vi "Kinect Demo.vi"() -> ()   [LabVIEW 2011]
uses:
  <vilib>/Utility/sysdir.llb/System Directory Type.ctl
  <vilib>/Platform/TimedLoop/XDataNode/XDataNode.xnode
  <vilib>/Platform/TimedLoop/XDataNode/nitl_modes.ctl
  <vilib>/Platform/TimedLoop/XDataNode/XDNodeRunTimeDep.lvlib
  <vilib>/Platform/TimedLoop/XDataNode/wakeup.ctl
  <vilib>/Platform/TimedLoop/XDataNode/timing_clust.ctl
  <vilib>/vision/NI_Vision_Development_Module.lvlib
panel:
  in  "Operation":T1(ring)=enum."Open"
  in  "Display Type":T2(ring)=enum."Baseline"
  in  "Post Extraction Limit":cluster{dbl, dbl}(slide)={0.0, 6291.456} scale=-3000.0..3000.0
  in  "stop 2":bool
  in  "# Frames in Average":i32=100
  in  "Start":bool
  in  "Zero Out Baseline":bool
  in  "Median Filter Size":i32=5 min=0 max=7
  in  "Divisor":sgl=0.5 min=0 max=1 step=0.1
  in  "name or relative path":string="Mouse Test"
  in  "Distance to Camera Visible":cluster{dbl, dbl}(slide)={0.0, 6291.456} scale=-32768.0..32768.0
  in  "Status":string
  out "Frame Display":T3(plugin-control)
  out "Image":T3(plugin-control)
  in  "stop":bool
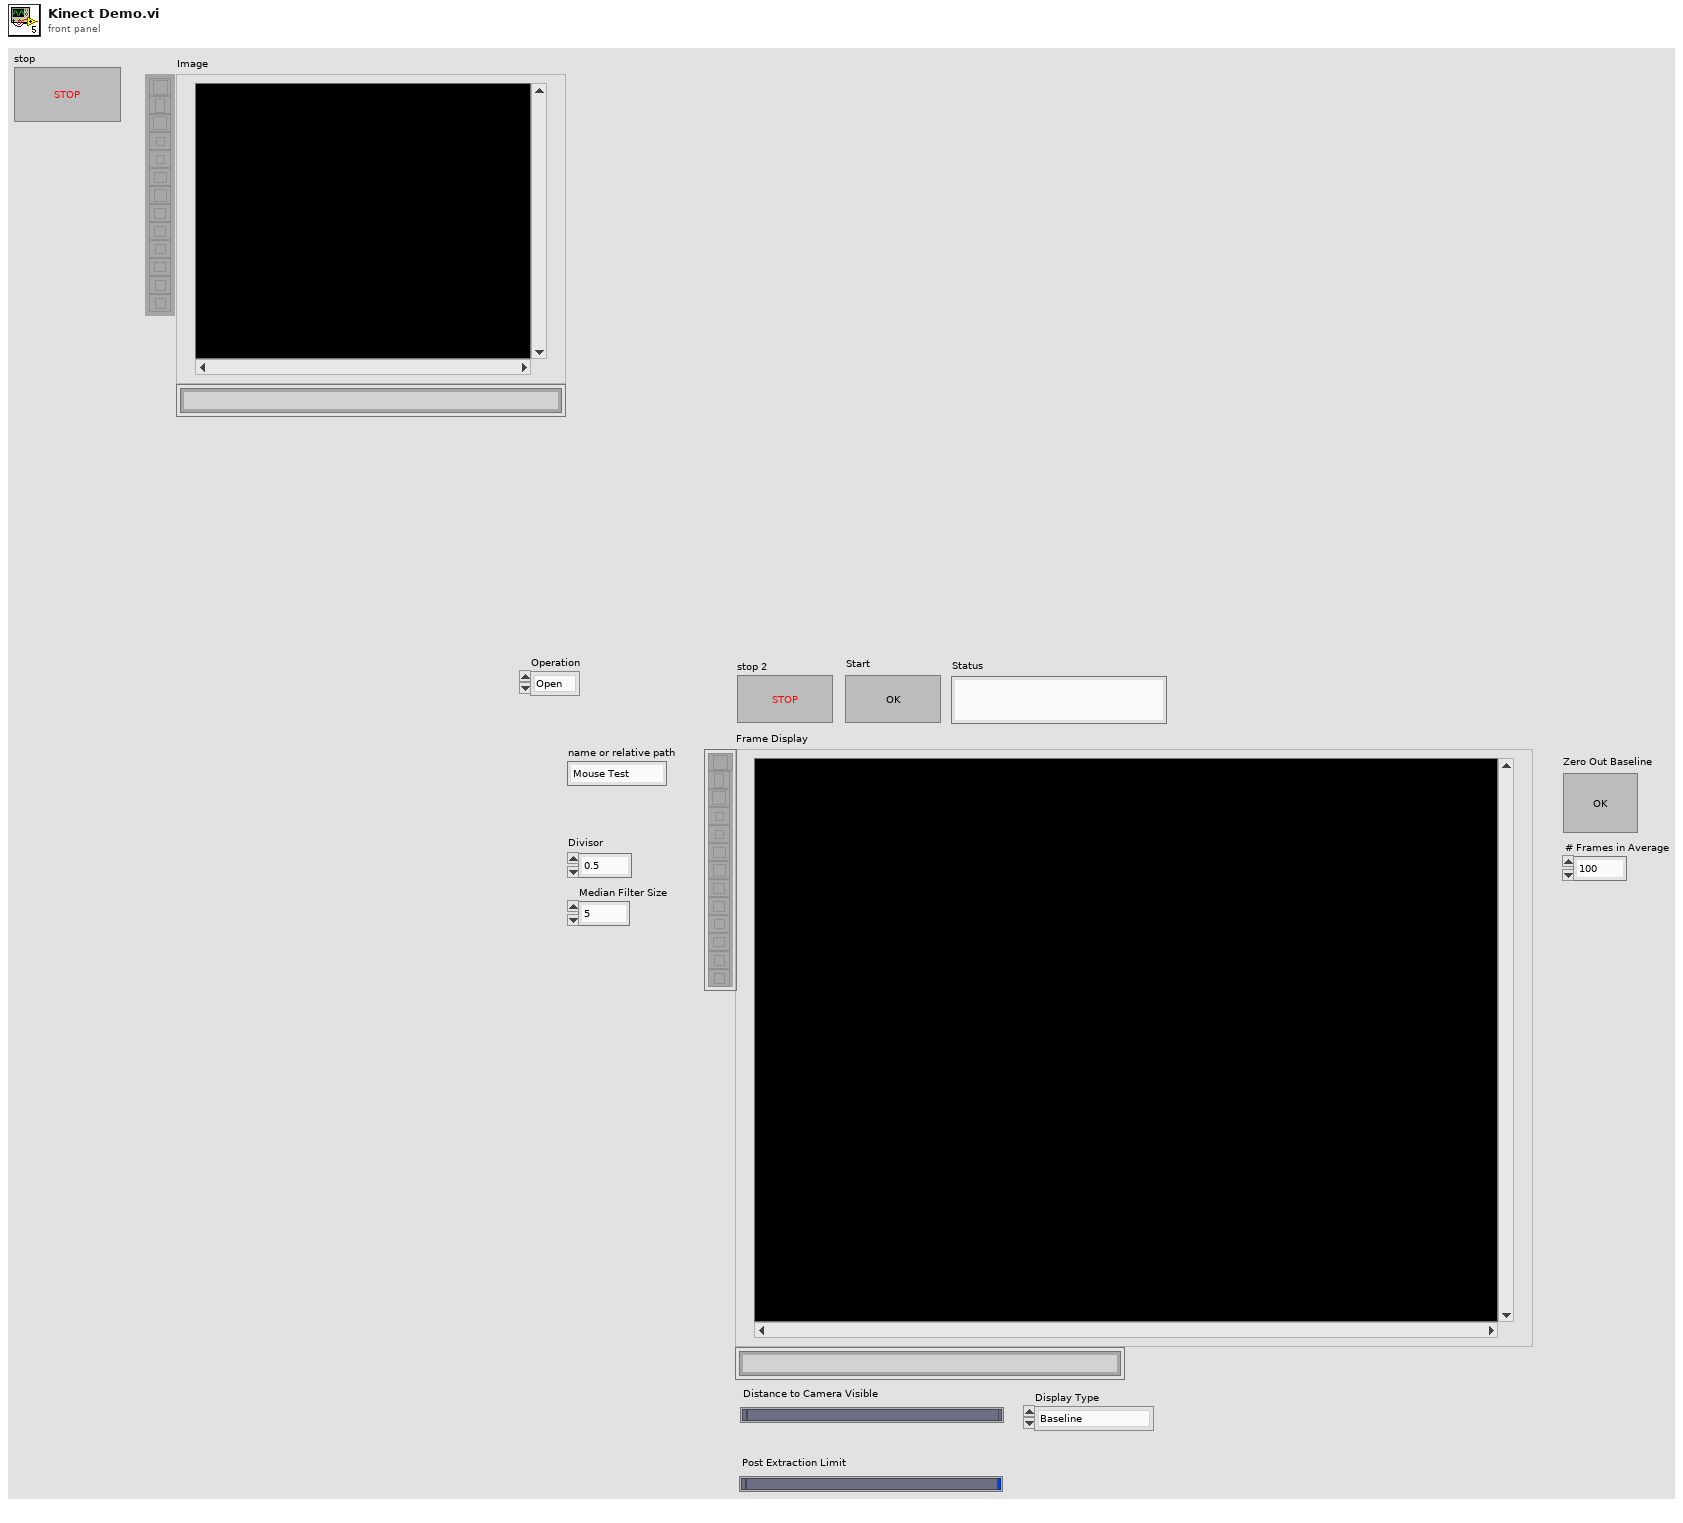
[diagram p1: front panel]
types:
  T1 = enum32{"AutoM", "Close", "Dilate", "Erode", "Gradient", "Gradient in", "Gradient out", "HitMiss", "Open", "PClose", "POpen", "Thick", "Thin"}
  T2 = enum16{"Raw Image", "Baseline", "Baseline Extracted"}
  T3 = typedef "IMAQ Image.ctl" = refnum<image>
  T4 = typedef "System Directory Type.ctl" = i32
  T5 = enum16{"Record", "Idle", "Acquire Background", "Stop"}
  T6 = typedef "XDNodeRunTimeDep.lvlib/timing_clust.ctl" = cluster{"Expected End [f-1]":u64, "Actual End [f-1]":u64, "Finished Late? [f-1]":bool, "Expected End [i-1]":u64, "Actual End [i-1]":u64, "Finished Late? [i-1]":bool, "Expected Start [i]":u64, "Actual Start [i]":u64, "Expected Start [f]":u64, "Actual Start [f]":u64, "Source Name":string, "Structure Name":string, "Period":i64, "Deadline":i64, "Offset":i64, "Start":i64, "Priority":i32, "Timeout":i32, "Mode":T7, "Wakeup Reason":T8, "Error":errorcluster, "Source Type":string, "Secondary Source Type":string, "Global End Time":u64, "Global Start Time":u64, "Frame Duration":u64, "Iteration Duration":u64, "Assigned CPU":i32, "I/O Scan Engine Mode":u32}
  T7 = typedef "XDNodeRunTimeDep.lvlib/nitl_modes.ctl" = enum32{"No Change", "Process missed periods, maintain original phase", "Discard missed periods, maintain original phase", "Process missed periods, ignore original phase", "Discard missed periods, ignore original phase"}
  T8 = typedef "XDNodeRunTimeDep.lvlib/wakeup.ctl" = enum32{"Normal", "Aborted", "Asynchronous wakeup", "Timing source error", "Timed loop error", "Timeout"}
  T9 = enum32{"Average", "Min", "Max", "Clear  if < ", "Clear  if < or =", "Clear  if =", "Clear  if > or =", "Clear  if >"}
  T10 = cluster{"Median Filter Size":i32, "Median Filter Size":i32, i32}
  T11 = typedef "Image Type" = u32
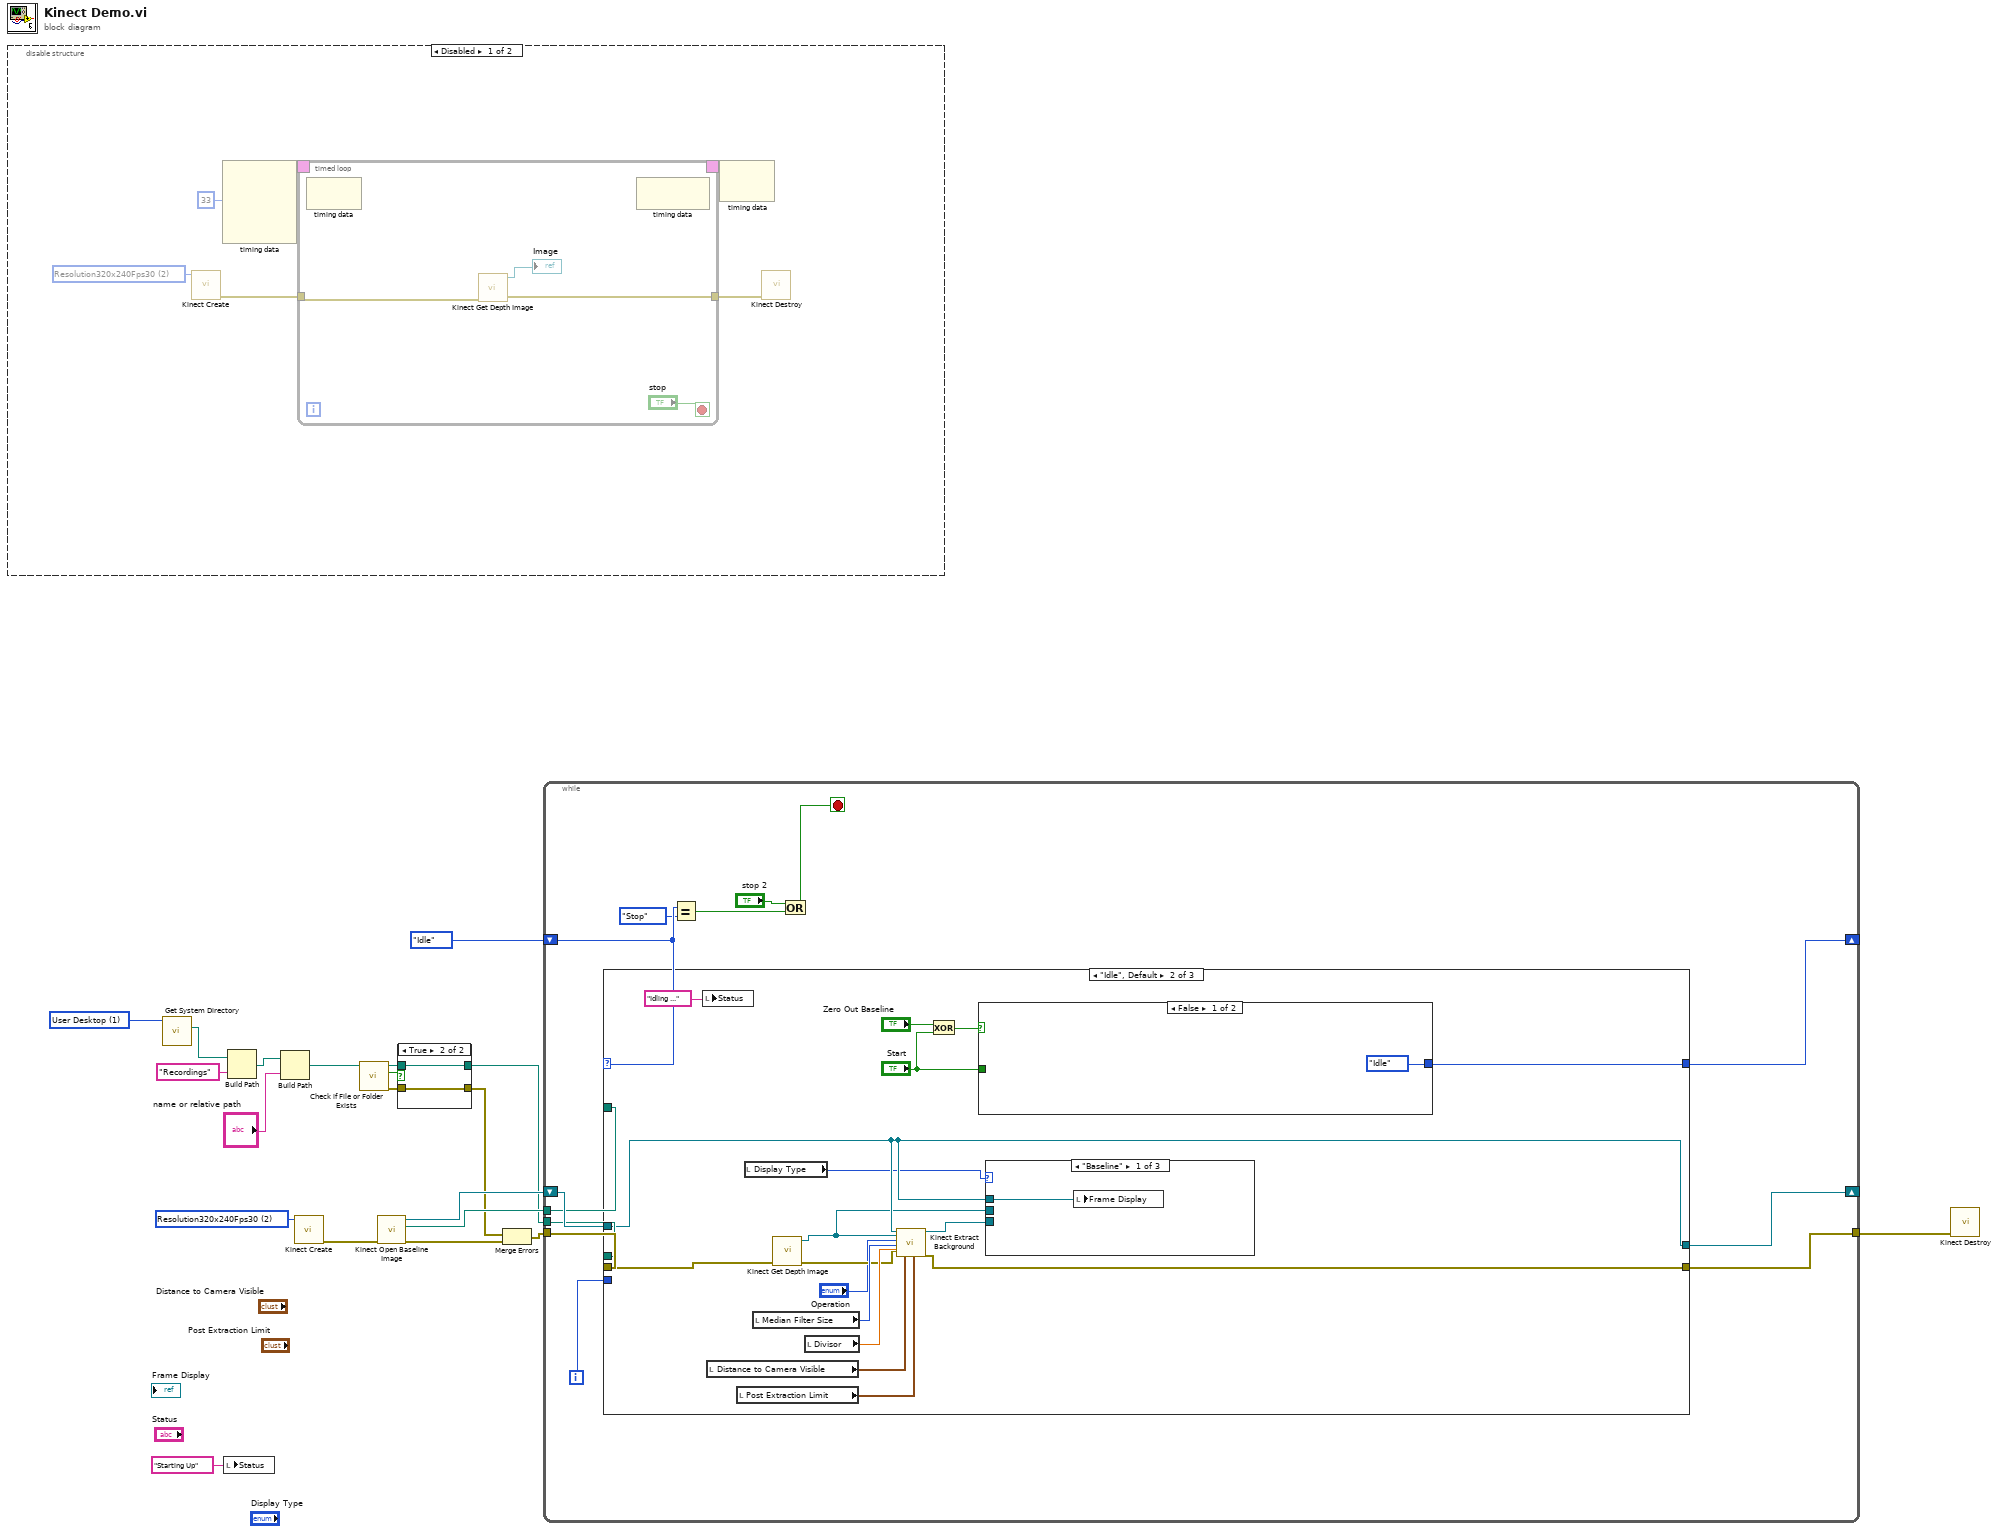
[diagram p0: block diagram]
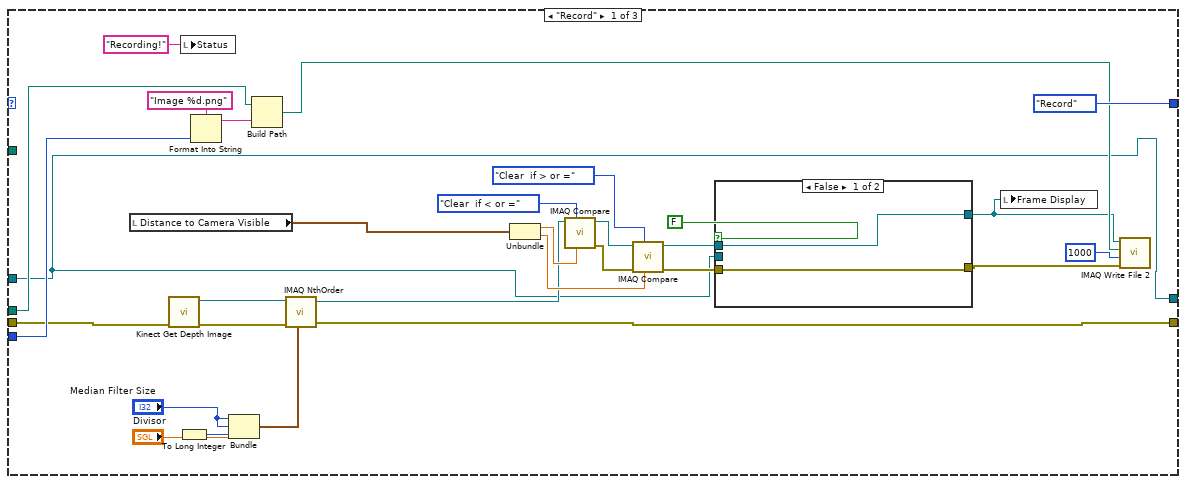
[diagram p2: hidden frame]
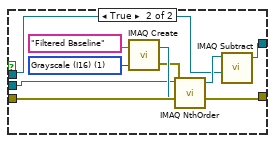
[diagram p3: hidden frame]
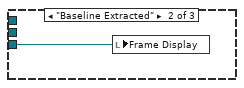
[diagram p4: hidden frame]
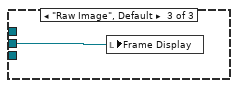
[diagram p5: hidden frame]
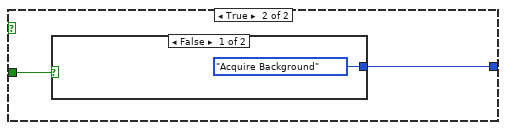
[diagram p6: hidden frame]
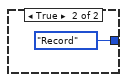
[diagram p7: hidden frame]
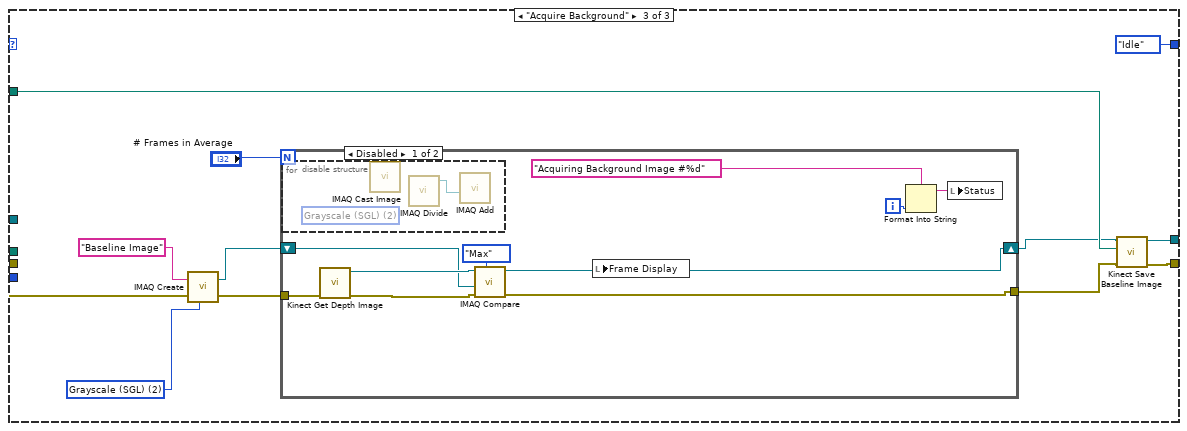
[diagram p8: hidden frame]
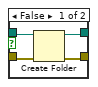
[diagram p11: hidden frame]
diagram:
  w16 = 2 items=["Undefined", "Resolution640x480Fps30", "Resolution320x240Fps30", "Resolution80x60Fps30"] ("Depth Format")
  w18 = T4 1 items=["User Home"=0, "User Desktop"=1, "User Documents"=2, "User Application Data"=3, "User Preferences"=4, "User Temporary"=5, "Public Documents"=6, "Public Application Data"=7, "Public Preferences"=8, "Public Cache"=13, "System Core Libraries"=9, "System Installed Libraries"=10, "Application Files"=11, "Boot Volume Root"=12] ("system directory type")
  n1 = disable-structure shown="Disabled" {
    frame Disabled {
      w23 = 2 items=["Undefined", "Resolution640x480Fps30", "Resolution320x240Fps30", "Resolution80x60Fps30"] ("Depth Format")
      n2 = call "Kinect Create.vi"("Depth Format"=w23) -> ("error out"=w24:errorcluster)  [unwired: 10 in]
      n3 = node-c288(i64 33 ("Period")) -> (w26:T6)  [unwired: 3 in]
      n4 = timed-loop {
        tunnel: [w29] -> w22
        tunnel: w24 -> [w28]
        timing: w26 -> [_]
        timing-out: [_] -> w25
        stop <- "stop" stop-if-true
        n5 = node-c288() -> ()  [unwired: 1 in, 1 out]
        n6 = call "Kinect Get Depth Image.vi"("error in (no error)"=w28) -> ("error out"=w29:errorcluster, "Depth Image"=→"Image":T3)  [unwired: 9 in]
        n7 = node-c288() -> ()  [unwired: 1 in, 1 out]
      }
      n8 = node-c288(w25) -> ()  [unwired: 1 out]
      n9 = call "Kinect Destroy.vi"("error in"=w22) -> ()  [unwired: 10 in, 1 out]
    }
    frame Enabled {
    }
  }
  n10 = call <vilib>:"Get System Directory.vi"("system directory type"=w18) -> ("system directory"=w17:path)  [unwired: 10 in]
  n11 = local write "Status"("Starting Up" ("Status")) -> ()
  n12 = Build Path(base path=w17, name or relative path="Recordings") -> (appended path=w11:path)
  n13 = Build Path(base path=w11, name or relative path="name or relative path") -> (appended path=w2:path)
  n14 = call "Kinect Create.vi"("Depth Format"=w16) -> ("error out"=w13:errorcluster)  [unwired: 10 in]
  n15 = call <vilib>:"Check if File or Folder Exists.vi"("path"=w2) -> ("error out"=w9:errorcluster, "file or folder exists?"=w7:bool, "dup path"=w8:path)  [unwired: 8 in]
  n16 = call "Kinect Open Baseline Image.vi"("error in (no error)"=w13) -> ("error out"=w4:errorcluster, "dup path"=w14:path, "Image Out"=w15:T3)  [unwired: 8 in]
  n17 = case shown="True" w7 {
    tunnel: w9 -> [w40 w41]
    tunnel: w8 -> [w39 w42]
    tunnel: [w37 w42] -> w6
    tunnel: [w38 w41] -> w3
    frame False {
      n18 = Create Folder(path (use dialog)=w39, error in=w40) -> (created path=w37:path, error out=w38:errorcluster)  [unwired: 1 in, 1 out]
    }
    frame True {
    }
  }
  n19 = Merge Errors(w3, w4) -> (w5:errorcluster)
  n20 = while {
    tunnel: w5 -> [w55]
    tunnel: [w54] -> w1
    shift-right: [w47] -> _
    shift-left: T5."Idle" -> [w49]
    shift-right: [w46] -> _
    shift-left: w15 -> [w53]
    tunnel: w14 -> [w45]
    tunnel: w6 -> [w43]
    i -> [w44]
    stop <- w51 stop-if-true
    n21 = case shown="\"Idle\", Default" w49 {
      tunnel: w55 -> [w65 w108 w129]
      tunnel: [w74 w103 w125] -> w54
      tunnel: w53 -> [w56 w100 _]
      tunnel: [T5."Record" w109 T5."Idle"] -> w47
      tunnel: [w56 w100 w126] -> w46
      tunnel: w45 -> [_ _ w123]
      tunnel: w44 -> [w71 _ _]
      tunnel: w43 -> [w70 _ _]
      frame "Record" {
        n22 = local read "Distance to Camera Visible"() -> (w77:cluster{dbl, dbl})
        n23 = call "Kinect Get Depth Image.vi"("error in (no error)"=w65) -> ("error out"=w66:errorcluster, "Depth Image"=w64:T3)  [unwired: 9 in]
        n24 = To Long Integer(number="Divisor") -> (32bit integer=w76:i32)
        n25 = local write "Status"("Recording!" ("Status")) -> ()
        n26 = Format Into String(format string="Image %d.png", w71) -> (resulting string=w72:string)  [unwired: 2 in, 1 out]
        n27 = Bundle("Median Filter Size"="Median Filter Size", "Median Filter Size"="Median Filter Size", w76) -> (w63:T10)  [unwired: 1 in]
        n28 = Build Path(base path=w70, name or relative path=w72) -> (appended path=w69:path)
        n29 = call "IMAQ NthOrder"("Image Src"=w64, "Size & Order #"=w63, "error in (no error)"=w66) -> ("Image Dst Out"=w62:T3, "error out"=w74:errorcluster)  [unwired: 4 in]
        n30 = Unbundle(w77) -> (w80:dbl, w79:dbl)
        n31 = call "IMAQ Compare"("Constant"=w80, "Operator"=T9."Clear  if < or =", "Image Src A"=w62) -> ("error out"=w82:errorcluster, "Image Dst Out"=w81:T3)  [unwired: 7 in]
        n32 = call "IMAQ Compare"("Constant"=w79, "Operator"=T9."Clear  if > or =", "error in (no error)"=w82, "Image Src A"=w81) -> ("error out"=w59:errorcluster, "Image Dst Out"=w61:T3)  [unwired: 6 in]
        n33 = case shown="False" FALSE {
          tunnel: w61 -> [w87 w88]
          tunnel: [w87 w96] -> w60
          tunnel: [w86 w95] -> w58
          tunnel: w59 -> [w86 w95]
          tunnel: w56 -> [_ w90]
          frame False {
          }
          frame True {
            w94 = T11 1 items=["Grayscale (U8)", "Grayscale (I16)", "Grayscale (SGL)", "Complex (CSG)", "RGB (U32)", "HSL (U32)", "RGB (U64)", "Grayscale (U16)"] ("Image Type")
            n34 = call "IMAQ Create"("Image Name"="Filtered Baseline", "Image Type"=w94) -> ("New Image"=w92:T3, "error out"=w91:errorcluster)  [unwired: 3 in]
            n35 = call "IMAQ NthOrder"("Image Src"=w90, "Image Dst"=w92, "error in (no error)"=w91) -> ("Image Dst Out"=w89:T3)  [unwired: 4 in, 1 out]
            n36 = call "IMAQ Subtract"("Image Src A"=w89, "Image Src B"=w88) -> ("Image Dst Out"=w96:T3)  [unwired: 5 in, 1 out]
          }
        }
        n37 = local write "Frame Display"(w60) -> ()
        n38 = call-poly "IMAQ Write File 2"("error in (no error)"=w58, "Image Quality"=u32 1000, "File Path"=w69, "Image"=w60) -> ()  [unwired: 6 in, 2 out]
      }
      frame "Idle", Default {
        n39 = local write "Status"("Idling ..." ("Status")) -> ()
        n40 = local read "Distance to Camera Visible"() -> (w104:cluster{dbl, dbl})
        n41 = local read "Post Extraction Limit"() -> (w102:cluster{dbl, dbl})
        n42 = local read "Display Type"() -> (w98:T2)
        n43 = local read "Median Filter Size"() -> (w107:i32)
        n44 = call "Kinect Get Depth Image.vi"("error in (no error)"=w108) -> ("error out"=w105:errorcluster, "Depth Image"=w99:T3)  [unwired: 9 in]
        n45 = local read "Divisor"() -> (w106:sgl)
        n46 = call "Kinect Extract Background.vi"("Background Image In"=w100, "Depth Image In"=w99, "Operation"="Operation", "Median Filter Size"=w107, "Divisor"=w106, "Distance to Camera Visible"=w104, "error in (no error)"=w105, "Post Proc Bounds"=w102) -> ("Processed Image Out"=w101:T3, "error out"=w103:errorcluster)  [unwired: 9 in, 1 out]
        n47 = Exclusive Or(1:"Start", 2:"Zero Out Baseline") -> (0:w111:bool)
        n48 = case shown="False" w111 {
          tunnel: "Start" -> [_ w119]
          tunnel: [T5."Idle" w118] -> w109
          frame False {
          }
          frame True {
            n49 = case shown="False" w119 {
              tunnel: [T5."Acquire Background" T5."Record"] -> w118
              frame False {
              }
              frame True {
              }
            }
          }
        }
        n50 = case shown="\"Baseline\"" w98 {
          tunnel: w101 -> [_ w115 _]
          tunnel: w100 -> [w114 _ _]
          tunnel: w99 -> [_ _ w116]
          frame "Baseline" {
            n51 = local write "Frame Display"(w114) -> ()
          }
          frame "Baseline Extracted" {
            n52 = local write "Frame Display"(w115) -> ()
          }
          frame "Raw Image", Default {
            n53 = local write "Frame Display"(w116) -> ()
          }
        }
      }
      frame "Acquire Background" {
        w132 = T11 2 items=["Grayscale (U8)", "Grayscale (I16)", "Grayscale (SGL)", "Complex (CSG)", "RGB (U32)", "HSL (U32)", "RGB (U64)", "Grayscale (U16)"] ("Image Type")
        n54 = call "IMAQ Create"("Image Name"="Baseline Image", "Image Type"=w132, "error in (no error)"=w129) -> ("New Image"=w131:T3, "error out"=w128:errorcluster)  [unwired: 2 in]
        n55 = for {
          N: "# Frames in Average" -> [_]
          tunnel: w128 -> [w140]
          shift-right: [w134] -> w122
          shift-left: w131 -> [w137]
          tunnel: [w135] -> w124
          i -> [w141]
          n56 = disable-structure shown="Disabled" {
            frame Disabled {
              (unwired) T11 2 items=["Grayscale (U8)", "Grayscale (I16)", "Grayscale (SGL)", "Complex (CSG)", "RGB (U32)", "HSL (U32)", "RGB (U64)", "Grayscale (U16)"] ("Image Type")
              n57 = call "IMAQ Cast Image"() -> ()  [unwired: 10 in, 2 out]
              n58 = call "IMAQ Divide"() -> ("Image Dst Out"=w144:T3)  [unwired: 7 in, 1 out]
              n59 = call "IMAQ Add"("Image Src B"=w144) -> ()  [unwired: 6 in, 2 out]
            }
            frame Enabled {
            }
          }
          n60 = call "Kinect Get Depth Image.vi"("error in (no error)"=w140) -> ("error out"=w136:errorcluster, "Depth Image"=w138:T3)  [unwired: 9 in]
          n61 = call "IMAQ Compare"("Operator"=T9."Max", "error in (no error)"=w136, "Image Src B"=w137, "Image Src A"=w138) -> ("error out"=w135:errorcluster, "Image Dst Out"=w134:T3)  [unwired: 6 in]
          n62 = local write "Frame Display"(w134) -> ()
          n63 = Format Into String(format string="Acquiring Background Image #%d" ("Status"), w141) -> (resulting string=w143:string)  [unwired: 2 in, 1 out]
          n64 = local write "Status"(w143) -> ()
        }
        n65 = call "Kinect Save Baseline Image.vi"("error in (no error)"=w124, "Baseline Image Path"=w123, "Baseline Image"=w122) -> ("error out"=w125:errorcluster, "Baseline Image Out"=w126:T3)  [unwired: 7 in]
      }
    }
    n66 = Equal?(x=w49, y=T5."Stop") -> (x = y?=w50:bool)
    n67 = Or(x="stop 2", y=w50) -> (x .or. y?=w51:bool)
  }
  n68 = call "Kinect Destroy.vi"("error in"=w1) -> ()  [unwired: 10 in, 1 out]
